vi "Module Name--constant.vi"() -> (3 "Module Name":string)   [LabVIEW 2021, in "Sequence Engine.lvlib"]
doc: "Return the name of the module that owns this VI. \n_____\nBased on DQMH Dev Tools: Project Template 7.1.1.1528."
uses:
  Sequence Engine.lvlib
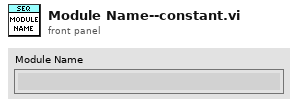
[diagram p1: front panel]
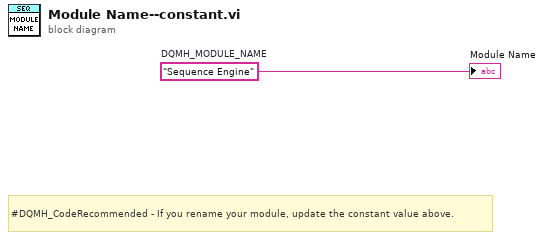
[diagram p0: block diagram]
diagram:
  w1 = "Sequence Engine"  # DQMH_MODULE_NAME
  # "#DQMH_CodeRecommended - If you rename your module, update the constant value above."
  "Module Name" <- w1
